vi "ResizeGenericGUIObject.vi"(4 "Force Aspect Ratio?":bool, 5 "Borders in Percent(T) or Pixels (F)":bool, 6 "Adjust":u16(ring) items=["Height", "Width", "Both"], 7 "Minimal":T1, 8 "error in (no error)":errorcluster, 9 "Borders":T2, 10 "generic class reference":refnum<vi>, 11 "PentaPanesGUI in":refnum<class "PentaPanes.lvclass">) -> (0 "error out":errorcluster, 2 "Class Name out":string, 3 "PentaPanesGUI out":refnum<class "PentaPanes.lvclass">)   [LabVIEW 2022 SP3, in "PentaPanesLibrary.lvlib" / "PentaPanes.lvclass"]
doc: "This VI resizes a labview control type of a supported controls."
uses:
  PentaPanes.lvclass
  BordersCluster.ctl
  <vilib>/Utility/miscctls.llb/LVBoundsTypeDef.ctl
panel:
  out "Class ID":u32
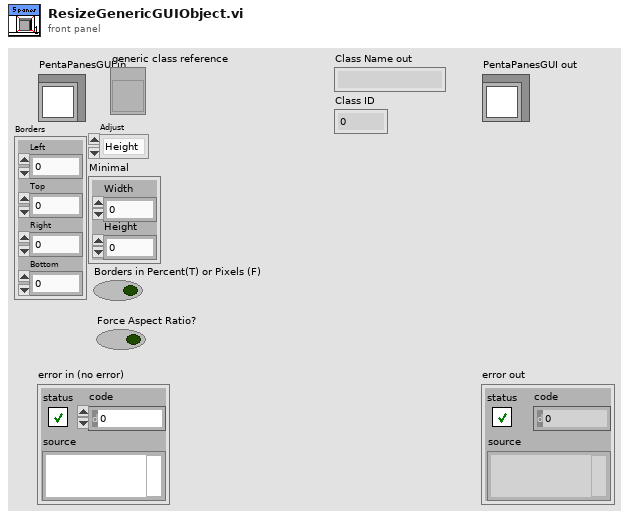
[diagram p1: front panel]
types:
  T1 = typedef "LVBoundsTypeDef.ctl" = cluster{"Width":i32, "Height":i32}
  T2 = typedef "PentaPanesLibrary.lvlib/PentaPanes.lvclass/BordersCluster.ctl" = cluster{"Left":i32, "Top":i32, "Right":i32, "Bottom":i32}
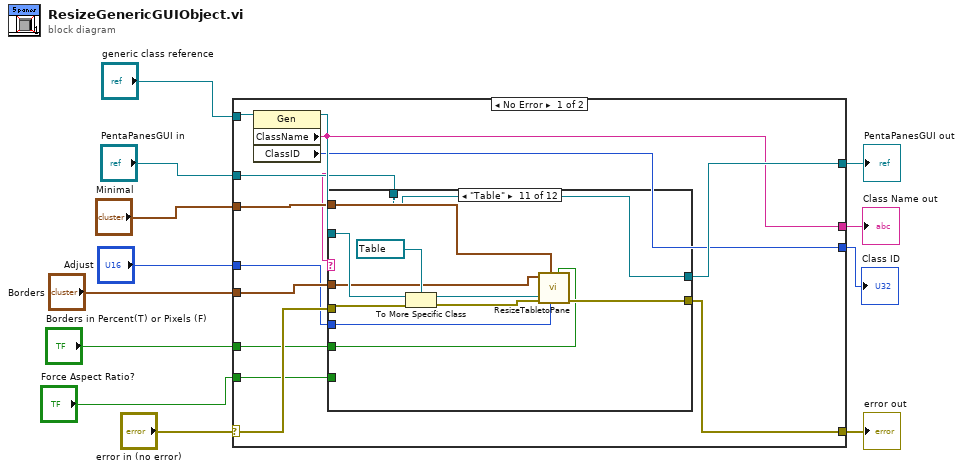
[diagram p0: block diagram]
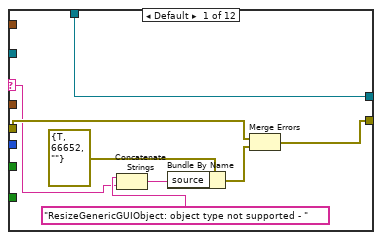
[diagram p2: hidden frame]
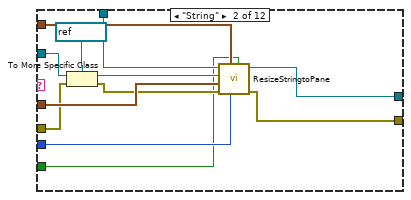
[diagram p3: hidden frame]
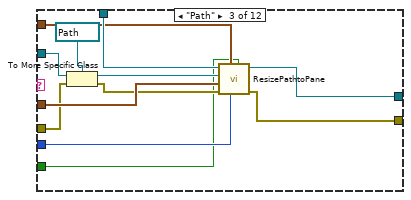
[diagram p4: hidden frame]
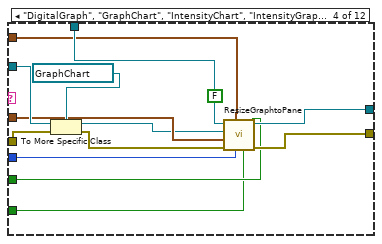
[diagram p5: hidden frame]
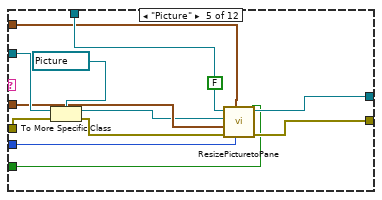
[diagram p6: hidden frame]
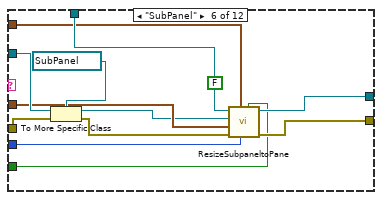
[diagram p7: hidden frame]
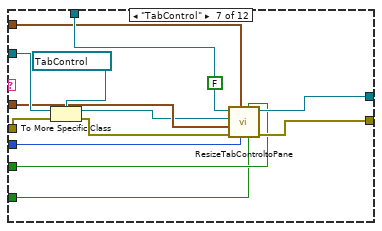
[diagram p8: hidden frame]
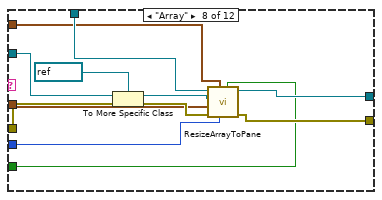
[diagram p9: hidden frame]
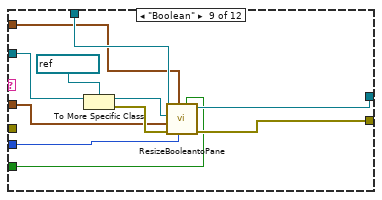
[diagram p10: hidden frame]
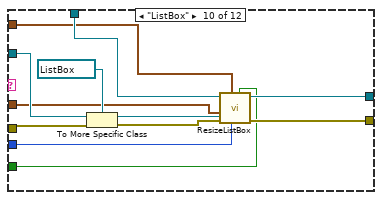
[diagram p11: hidden frame]
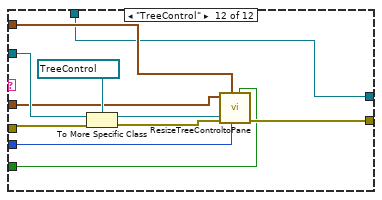
[diagram p12: hidden frame]
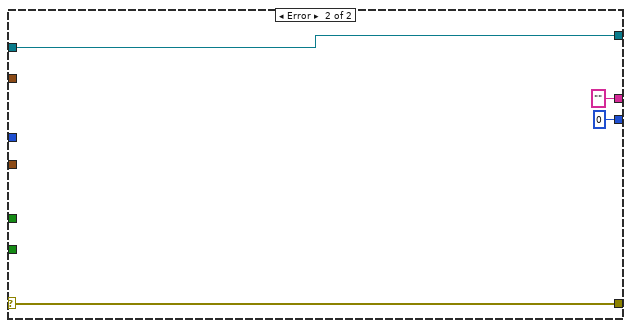
[diagram p13: hidden frame]
diagram:
  n1 = case shown="No Error" "error in (no error)" {
    selector: "error in (no error)" -> [w20 w168]
    tunnel: [w19 w168] -> w11
    tunnel: [w22 w167] -> w9
    tunnel: "PentaPanesGUI in" -> [w23 w167]
    tunnel: "generic class reference" -> [w25 _]
    tunnel: "Borders" -> [w21 _]
    tunnel: "Adjust" -> [w18 _]
    tunnel: "Minimal" -> [w17 _]
    tunnel: [w16 "" ("ClassName")] -> w4
    tunnel: [w15 u32 0 ("ClassID")] -> w3
    tunnel: "Borders in Percent(T) or Pixels (F)" -> [w14 _]
    tunnel: "Force Aspect Ratio?" -> [w13 _]
    frame No Error {
      n2 = property class="Gen"(reference=w25) -> (reference out=w24:refnum<vi>, "ClassName"=w16:string, "ClassID"=w15:u32)  [unwired: 1 in, 1 out]
      n3 = case shown="\"Table\"" w16 {
        selector: w16 -> [w27 _ _ _ _ _ _ _ _ _ _ _]
        tunnel: w24 -> [_ w44 w56 w70 w82 w94 w107 w119 w130 w142 w153 w164]
        tunnel: w23 -> [w33 w45 w57 w68 w80 w86 w99 w117 w124 w139 w143 w154]
        tunnel: [w33 w40 w52 w67 w79 w84 w97 w116 w125 w138 w143 w154] -> w22
        tunnel: w21 -> [_ w41 w53 w66 w78 w88 w101 w112 w123 w135 w148 w159]
        tunnel: w20 -> [w32 w36 w48 w63 w75 w92 w105 w115 _ w134 w147 w158]
        tunnel: [w31 w39 w51 w62 w74 w90 w103 w113 w126 w136 w149 w160] -> w19
        tunnel: w18 -> [_ w37 w49 w61 w73 w89 w102 w110 w122 w132 w145 w156]
        tunnel: w17 -> [_ w38 w50 w60 w72 w85 w98 w109 w121 w133 w146 w157]
        tunnel: w14 -> [_ w34 w46 w59 w71 w83 w96 w108 w120 w131 w144 w155]
        tunnel: w13 -> [_ _ _ w58 _ _ w95 _ _ _ _ _]
        frame Default {
          n4 = Concatenate Strings("ResizeGenericGUIObject: object type not supported - ", w27) -> (w26:string)
          n5 = Bundle By Name(cluster=errorcluster {"status"=TRUE, "code"=66652, "source"=""} ("error constant"), "source"=w26) -> (w30:errorcluster)
          n6 = Merge Errors(w32, w30) -> (w31:errorcluster)
        }
        frame "String" {
          n7 = To More Specific Class(target class=refnum<vi> refnum ("String"), reference=w44, error in=w36) -> (specific class reference=w42:refnum<vi>, error out=w35:errorcluster)
          n8 = call "ResizeStringtoPane.vi"("Borders in Percent(T) or Pixels (F)"=w34, "Adjust"=w37, "Minimal"=w38, "error in (no error)"=w35, "Borders"=w41, "String"=w42, "PentaPanesGUI in"=w45) -> ("error out"=w39:errorcluster, "PentaPanesGUI out"=w40:refnum<class "PentaPanes.lvclass">)  [unwired: 3 in]
        }
        frame "Path" {
          n9 = To More Specific Class(target class=refnum<vi> refnum ("String"), reference=w56, error in=w48) -> (specific class reference=w54:refnum<vi>, error out=w47:errorcluster)
          n10 = call "ResizePathtoPane.vi"("Borders in Percent(T) or Pixels (F)"=w46, "Adjust"=w49, "Minimal"=w50, "error in (no error)"=w47, "Borders"=w53, "Path"=w54, "PentaPanesGUI in"=w57) -> ("error out"=w51:errorcluster, "PentaPanesGUI out"=w52:refnum<class "PentaPanes.lvclass">)  [unwired: 3 in]
        }
        frame "DigitalGraph", "GraphChart", "IntensityChart", "IntensityGraph", "MixedSignalGraph", "WaveformChart", "WaveformGraph", "XYGraph" {
          (unwired) FALSE ("Borders in Percent(T) or Pixels (F)")
          n11 = To More Specific Class(target class=refnum<vi> refnum ("XY Graph"), reference=w70, error in=w63) -> (specific class reference=w65:refnum<vi>, error out=w64:errorcluster)
          n12 = call "ResizeGraphtoPane.vi"("Force aspect ratio?"=w58, "Borders in Percent(T) or Pixels (F)"=w59, "Adjust"=w61, "Minimal"=w60, "error in (no error)"=w64, "Borders"=w66, "Graph Chart"=w65, "PentaPanesGUI in"=w68) -> ("error out"=w62:errorcluster, "PentaPanesGUI out"=w67:refnum<class "PentaPanes.lvclass">)  [unwired: 2 in]
        }
        frame "Picture" {
          (unwired) FALSE ("Borders in Percent(T) or Pixels (F)")
          n13 = To More Specific Class(target class=refnum<vi> refnum ("XY Graph"), reference=w82, error in=w75) -> (specific class reference=w77:refnum<vi>, error out=w76:errorcluster)
          n14 = call "ResizePicturetoPane.vi"("Borders in Percent(T) or Pixels (F)"=w71, "Adjust"=w73, "Minimal"=w72, "error in (no error)"=w76, "Borders"=w78, "Picture"=w77, "PentaPanesGUI in"=w80) -> ("error out"=w74:errorcluster, "PentaPanesGUI out"=w79:refnum<class "PentaPanes.lvclass">)  [unwired: 3 in]
        }
        frame "SubPanel" {
          (unwired) FALSE ("Borders in Percent(T) or Pixels (F)")
          n15 = To More Specific Class(target class=refnum<vi> refnum ("XY Graph"), reference=w94, error in=w92) -> (specific class reference=w87:refnum<vi>, error out=w91:errorcluster)
          n16 = call "ResizeSubpaneltoPane.vi"("Borders in Percent(T) or Pixels (F)"=w83, "Adjust"=w89, "Minimal"=w85, "error in (no error)"=w91, "Borders"=w88, "SubPanel"=w87, "PentaPanesGUI in"=w86) -> ("error out"=w90:errorcluster, "PentaPanesGUI out"=w84:refnum<class "PentaPanes.lvclass">)  [unwired: 3 in]
        }
        frame "TabControl" {
          (unwired) FALSE ("Borders in Percent(T) or Pixels (F)")
          n17 = To More Specific Class(target class=refnum<vi> refnum ("XY Graph"), reference=w107, error in=w105) -> (specific class reference=w100:refnum<vi>, error out=w104:errorcluster)
          n18 = call "ResizeTabControltoPane.vi"("Force aspect ratio?"=w95, "Borders in Percent(T) or Pixels (F)"=w96, "Adjust"=w102, "Minimal"=w98, "error in (no error)"=w104, "Borders"=w101, "TabControl"=w100, "PentaPanesGUI in"=w99) -> ("error out"=w103:errorcluster, "PentaPanesGUI out"=w97:refnum<class "PentaPanes.lvclass">)  [unwired: 2 in]
        }
        frame "Array" {
          n19 = To More Specific Class(target class=refnum<vi> refnum ("Array"), reference=w119, error in=w115) -> (specific class reference=w111:refnum<vi>, error out=w114:errorcluster)
          n20 = call "ResizeArrayToPane.vi"("Borders in Percent(T) or Pixels (F)"=w108, "Adjust"=w110, "Minimal"=w109, "error in (no error)"=w114, "Borders"=w112, "Array"=w111, "PentaPanesGUI in"=w117) -> ("error out"=w113:errorcluster, "PentaPanesGUI out"=w116:refnum<class "PentaPanes.lvclass">)  [unwired: 3 in]
        }
        frame "Boolean" {
          n21 = To More Specific Class(target class=refnum<vi> refnum ("Boolean"), reference=w130) -> (specific class reference=w128:refnum<vi>, error out=w127:errorcluster)  [unwired: 1 in]
          n22 = call "ResizeBooleantoPane.vi"("Borders in Percent(T) or Pixels (F)"=w120, "Adjust"=w122, "Minimal"=w121, "error in (no error)"=w127, "Borders"=w123, "Boolean"=w128, "PentaPanesGUI in"=w124) -> ("error out"=w126:errorcluster, "PentaPanesGUI out"=w125:refnum<class "PentaPanes.lvclass">)  [unwired: 3 in]
        }
        frame "ListBox" {
          n23 = To More Specific Class(target class=refnum<vi> refnum ("Listbox"), reference=w142, error in=w134) -> (specific class reference=w140:refnum<vi>, error out=w137:errorcluster)
          n24 = call "ResizeListBox.vi"("Borders in Percent(T) or Pixels (F)"=w131, "Adjust"=w132, "Minimal"=w133, "error in (no error)"=w137, "Borders"=w135, "Listbox"=w140, "PentaPanesGUI in"=w139) -> ("error out"=w136:errorcluster, "PentaPanesGUI out"=w138:refnum<class "PentaPanes.lvclass">)  [unwired: 3 in]
        }
        frame "Table" {
          n25 = To More Specific Class(target class=refnum<vi> refnum ("Listbox"), reference=w153, error in=w147) -> (specific class reference=w151:refnum<vi>, error out=w150:errorcluster)
          n26 = call "ResizeTabletoPane.vi"("Borders in Percent(T) or Pixels (F)"=w144, "Adjust"=w145, "Minimal"=w146, "error in (no error)"=w150, "Table"=w151, "Borders"=w148) -> ("error out"=w149:errorcluster)  [unwired: 5 in]
        }
        frame "TreeControl" {
          n27 = To More Specific Class(target class=refnum<vi> refnum ("Listbox"), reference=w164, error in=w158) -> (specific class reference=w162:refnum<vi>, error out=w161:errorcluster)
          n28 = call "ResizeTreeControltoPane.vi"("Borders in Percent(T) or Pixels (F)"=w155, "Adjust"=w156, "Minimal"=w157, "error in (no error)"=w161, "Table"=w162, "Borders"=w159) -> ("error out"=w160:errorcluster)  [unwired: 5 in]
        }
      }
    }
    frame Error {
    }
  }
  "error out" <- w11
  "PentaPanesGUI out" <- w9
  "Class Name out" <- w4
  "Class ID" <- w3
